vi "Swerve Wheel.vi"(2 "Wheel":T1(ring), 4 "Inputs":dbl[](array[numeric])) -> (0 "Speed":dbl)   [LabVIEW 2013]
doc: "Used within Swerve Drive.vi.\nControls an individual wheel."
uses:
  <vilib>/addons/control/pid/pid.llb/PID (DBL).vi
  <vilib>/addons/control/pid/NI_PID_pid.lvlib
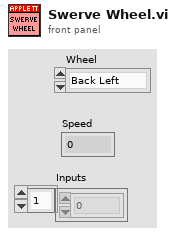
[diagram p1: front panel]
types:
  T1 = enum16{"Back Left", "Back Right", "Front Left", "Front Right"}
  T2 = enum16{"Z", "Y", "X", "Rot. Point X", "Rot. Point Y", "Width/2", "Max", "Length/2"}
  T3 = enum16{"Z Axis", "Y", "X", "Rot. Point X", "Rot. Point Y", "Width/2", "Max", "Length/2"}
  T4 = cluster{"proportional gain (Kc)":dbl, "integral time (Ti, min)":dbl, "derivative time (Td, min)":dbl}
  T5 = typedef "WPI_AnalogChannelDevRef.ctl" = cluster{"DevStatus":errorcluster, "Analog Module":T6, "Analog Channel":T7}
  T6 = typedef "FPGA_TypedefAnalogModule.ctl" = enum16{"Analog Module 1", "Analog Module 2"}
  T7 = typedef "FPGA_AIChannel.ctl" = enum8{"AI 1", "AI 2", "AI 3", "AI 4", "AI 5", "AI 6", "AI 7", "AI 8", "Invalid"}
  T8 = typedef "WPI_MotorControlDeviceRef.ctl" = cluster{"DeviceStatus":errorcluster, "Type":enum16{"PWM", "CAN"}, "PWM":cluster{"Digital Module":T9, "PWM Channel":T10, "DeadBand":T11}, "CAN":cluster{"Device Number":u8, "Control Mode":T12, "Semaphore":T13, "Max Vout":dbl}, "Invert":bool, "TransformRef":T14, "InvTransformRef":T14}
  T9 = typedef "FPGA_TypedefDigitalModule.ctl" = enum16{"Digital Module 1", "Digital Module 2"}
  T10 = typedef "FPGA_DIOPWMChannel.ctl" = enum8{"PWM 1", "PWM 2", "PWM 3", "PWM 4", "PWM 5", "PWM 6", "PWM 7", "PWM 8", "PWM 9", "PWM 10", "Invalid"}
  T11 = typedef "WPI_PWMDeadband.ctl" = cluster{"Name":string, "maxPositivePwm":i32, "minPositivePwm":i32, "centerPwm":i32, "maxNegativePwm":i32, "minNegativePwm":i32, "angularRange":u16}
  T12 = typedef "WPI_CANJaguar_ControlMode.ctl" = enum8{"Percent VBus", "Current", "Speed", "Position", "Voltage"}
  T13 = typedef "Semaphore RefNum" = refnum<k1>
  T14 = typedef "WPI_PWMTransform_ConPane.ctl" = refnum<vi>
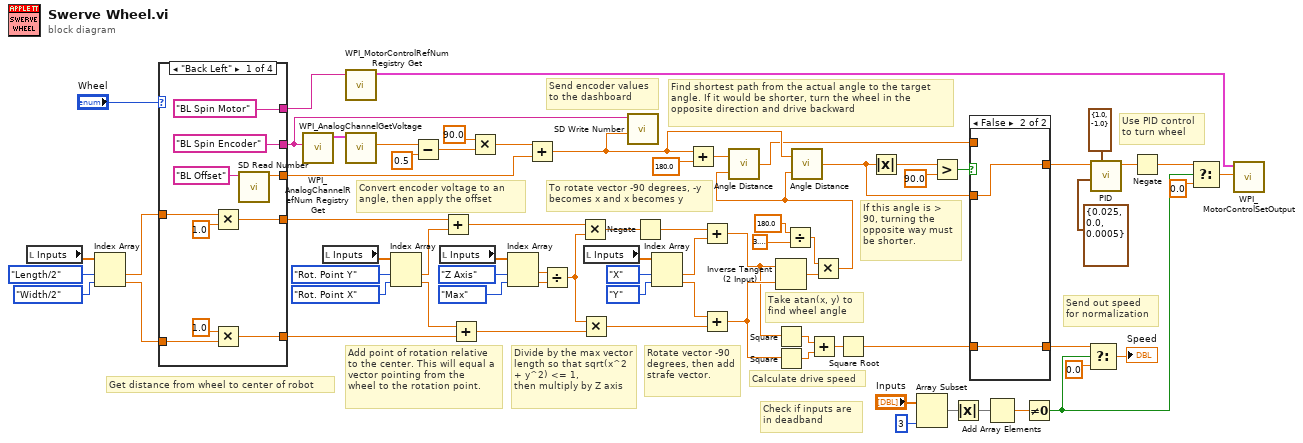
[diagram p0: block diagram]
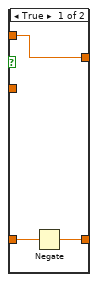
[diagram p2: hidden frame]
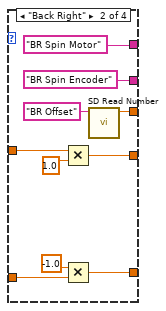
[diagram p3: hidden frame]
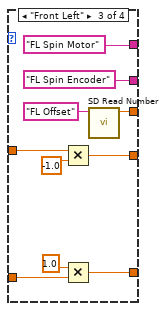
[diagram p4: hidden frame]
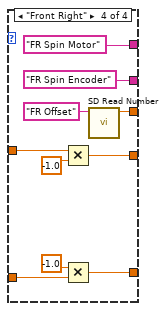
[diagram p5: hidden frame]
diagram:
  # "Send encoder values \nto the dashboard"
  # "To rotate vector -90 degrees, -y becomes x and x becomes y"
  # "Divide by the max vector length so that sqrt(x^2 + y^2) <= 1,\nthen multiply by Z axis"
  # "Add point of rotation relative to the center. This will equal a vector pointing from the\nwheel to the rotation point."
  # "Send out speed\nfor normalization"
  # "Check if inputs are\nin deadband"
  # "Convert encoder voltage to an angle, then apply the offset"
  # "If this angle is > 90, turning the opposite way must be shorter."
  # "Use PID control\nto turn wheel"
  # "Find shortest path from the actual angle to the target angle. If it would be shorter, turn the wheel in the opposite direction and drive backward"
  # "Take atan(x, y) to find wheel angle"
  # "Calculate drive speed"
  # "Rotate vector -90 degrees, then add strafe vector."
  # "Get distance from wheel to center of robot"
  n1 = local read "Inputs"() -> (w11:dbl[])
  n2 = Index Array(array=w11, index #1=T2."Length/2", index #2=T2."Width/2") -> (element #1=w9:dbl, element #2=w8:dbl)
  n3 = case shown="\"Back Left\"" "Wheel" {
    tunnel: ["BL Spin Encoder" "BR Spin Encoder" "FL Spin Encoder" "FR Spin Encoder"] -> w38
    tunnel: ["BL Spin Motor" "BR Spin Motor" "FL Spin Motor" "FR Spin Motor"] -> w59
    tunnel: [w81 w91 w101 w111] -> w49
    tunnel: w9 -> [w79 w89 w99 w109]
    tunnel: w8 -> [w77 w87 w97 w107]
    tunnel: [w76 w86 w96 w106] -> w35
    tunnel: [w75 w85 w95 w105] -> w31
    frame "Back Left" {
      n4 = Multiply(x=w79, y=1.0) -> (x*y=w76:dbl)
      n5 = Multiply(x=1.0 ("y"), y=w77) -> (x*y=w75:dbl)
      n6 = call <vilib>:"SD Read Number.vi"("Name"="BL Offset") -> ("Numeric"=w81:dbl)  [unwired: 8 in, 2 out]
    }
    frame "Back Right" {
      n7 = Multiply(x=w89, y=1.0) -> (x*y=w86:dbl)
      n8 = Multiply(x=-1.0 ("y"), y=w87) -> (x*y=w85:dbl)
      n9 = call <vilib>:"SD Read Number.vi"("Name"="BR Offset") -> ("Numeric"=w91:dbl)  [unwired: 8 in, 2 out]
    }
    frame "Front Left" {
      n10 = Multiply(x=w99, y=-1.0) -> (x*y=w96:dbl)
      n11 = Multiply(x=1.0 ("y"), y=w97) -> (x*y=w95:dbl)
      n12 = call <vilib>:"SD Read Number.vi"("Name"="FL Offset") -> ("Numeric"=w101:dbl)  [unwired: 8 in, 2 out]
    }
    frame "Front Right" {
      n13 = Multiply(x=w109, y=-1.0) -> (x*y=w106:dbl)
      n14 = Multiply(x=-1.0 ("y"), y=w107) -> (x*y=w105:dbl)
      n15 = call <vilib>:"SD Read Number.vi"("Name"="FR Offset") -> ("Numeric"=w111:dbl)  [unwired: 8 in, 2 out]
    }
  }
  n16 = call <vilib>:"WPI_AnalogChannelRefNum Registry Get.vi"("refnum name"=w38) -> ("AIDeviceRef"=w54:T5)  [unwired: 9 in, 1 out]
  n17 = local read "Inputs"() -> (w33:dbl[])
  n18 = call <vilib>:"WPI_MotorControlRefNum Registry Get.vi"("refnum name"=w59) -> ("MotorControlDevRef"=w72:T8)  [unwired: 9 in, 1 out]
  n19 = call <vilib>:"WPI_AnalogChannelGetVoltage.vi"("AIDeviceRef"=w54) -> ("Voltage"=w53:dbl)  [unwired: 8 in, 2 out]
  n20 = Index Array(array=w33, index #1=T2."Rot. Point Y", index #2=T2."Rot. Point X") -> (element #1=w29:dbl, element #2=w30:dbl)
  n21 = Subtract(x=w53, y=0.5) -> (x-y=w52:dbl)
  n22 = local read "Inputs"() -> (w27:dbl[])
  n23 = Add(x=w35, y=w29) -> (x+y=w4:dbl)
  n24 = Add(x=w30, y=w31) -> (x+y=w23:dbl)
  n25 = Multiply(x=90.0 ("y"), y=w52) -> (x*y=w50:dbl)
  n26 = Index Array(array=w27, index #1=T3."Z Axis", index #2=T2."Max") -> (element #1=w24:dbl, element #2=w25:dbl)
  n27 = Add(x=w50, y=w49) -> (x+y=w2:dbl)
  n28 = Divide(x=w24, y=w25) -> (x/y=w22:dbl)
  n29 = Multiply(x=w4, y=w22) -> (x*y=w6:dbl)
  n30 = Multiply(x=w22, y=w23) -> (x*y=w17:dbl)
  n31 = local read "Inputs"() -> (w20:dbl[])
  n32 = call <vilib>:"SD Write Number.vi"("Numeric"=w2, "Name"=w38) -> ()  [unwired: 8 in, 2 out]
  n33 = Negate(x=w6) -> (-x=w5:dbl)
  n34 = Index Array(array=w20, index #1=T2."X", index #2=T2."Y") -> (element #1=w15:dbl, element #2=w16:dbl)
  n35 = Add(x=w2, y=180.0 ("f")) -> (x+y=w45:dbl)
  n36 = Add(x=w5, y=w15) -> (x+y=w13:dbl)
  n37 = Add(x=w16, y=w17) -> (x+y=w14:dbl)
  n38 = Inverse Tangent (2 Input)(1:w14, 2:w13) -> (0:w70:dbl)
  n39 = Square(x=w13) -> (x^2=w18:dbl)
  n40 = Square(x=w14) -> (x^2=w69:dbl)
  n41 = Divide(x=180.0 ("y"), y=3.141592653589793) -> (x/y=w67:dbl)
  n42 = Add(x=w18, y=w69) -> (x+y=w68:dbl)
  n43 = Multiply(x=w67, y=w70) -> (x*y=w7:dbl)
  n44 = call "Angle Distance.vi"("target angle"=w7, "current angle"=w45) -> ("distance"=w1:dbl)
  n45 = call "Angle Distance.vi"("target angle"=w7, "current angle"=w2) -> ("distance"=w61:dbl)
  n46 = Square Root(x=w68) -> (sqrt(x)=w60:dbl)
  n47 = Absolute Value(x=w61) -> (abs(x)=w62:dbl)
  n48 = Array Subset(array="Inputs", length=3) -> (w44:dbl[])  [unwired: 1 in]
  n49 = Greater?(x=w62, y=90.0) -> (0:w40:bool)
  n50 = Absolute Value(x=w44) -> (abs(x)=w36:dbl[])
  n51 = case shown="False" w40 {
    tunnel: w1 -> [w115 _]
    tunnel: w61 -> [_ w119]
    tunnel: [w116 w118] -> w43
    tunnel: w60 -> [w117 w118]
    tunnel: [w115 w119] -> w56
    frame True {
      n52 = Negate(x=w117) -> (-x=w116:dbl)
    }
    frame False {
    }
  }
  n53 = Add Array Elements(numeric array=w36) -> (sum=w71:dbl)
  n54 = Not Equal To 0?(x=w71) -> (x != 0?=w39:bool)
  n55 = Select(t=w43, s=w39, f=0.0) -> (s? t:f=→"Speed":dbl)
  n56 = call-poly <vilib>:"PID.vi"("output range"=cluster{"output high":dbl, "output low":dbl} {"output high"=1.0, "output low"=-1.0}, "PID gains"=T4 {"proportional gain (Kc)"=0.025, "integral time (Ti, min)"=0.0, "derivative time (Td, min)"=0.0005}, "setpoint"=w56) -> ("output"=w47:dbl)  [unwired: 7 in, 1 out]
  n57 = Negate(x=w47) -> (-x=w37:dbl)
  n58 = Select(t=w37, s=w39, f=0.0) -> (s? t:f=w48:dbl)
  n59 = call <vilib>:"WPI_MotorControlSetOutput.vi"("Output"=w48, "MotorControlDevRef"=w72) -> ()  [unwired: 7 in, 3 out]
